vi "FreshTableDisplay.vi"(8 "error in (no error)":errorcluster, 10 "IndexDelta":i32, 11 "AdvanceTable in":refnum<class "AdvanceTable.lvclass">) -> (0 "error out":errorcluster, 3 "AdvanceTable out":refnum<class "AdvanceTable.lvclass">)   [LabVIEW 2015, in "ActorManagement.lvlib" / "AdvanceTable.lvclass"]
uses:
  AdvanceTable.lvclass
  AdvanceTable.lvclass/AdvanceTable.ctl
  Config/g_tabSetting.vi
  ActorManagement.lvlib
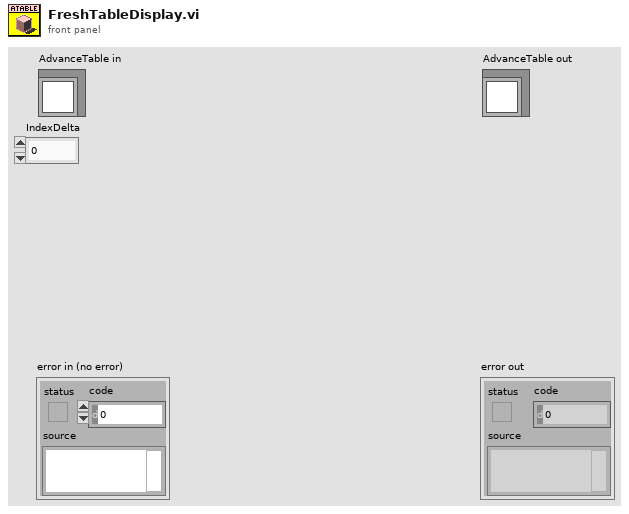
[diagram p1: front panel]
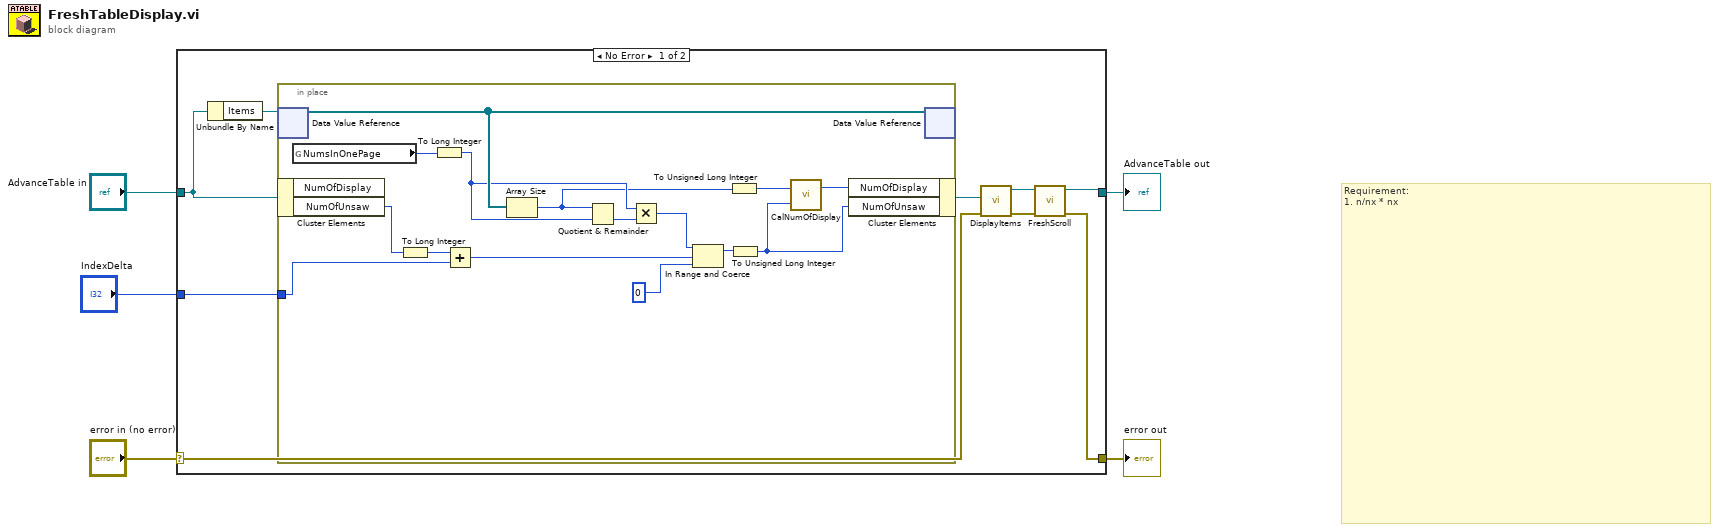
[diagram p0: block diagram]
diagram:
  # "Requirement:\n1. n/nx * nx"
  n1 = case shown="No Error" "error in (no error)" {
    selector: "error in (no error)" -> [w10 w31]
    tunnel: [w7 w31] -> w4
    tunnel: [w6 w30] -> w2
    tunnel: "AdvanceTable in" -> [w13 w30]
    tunnel: "IndexDelta" -> [w14 _]
    frame No Error {
      n2 = Unbundle By Name(w13) -> ("Items"=w12:refnum<data-value>)
      n3 = in-place {
        in-place-border: w14 -> [w26]
        n4 = in-place-dvr #1(w12) -> (w27:refnum<class "TableItem.lvclass">[])  [unwired: 1 out]
        n5 = in-place-cluster #2(w13) -> ("NumOfUnsaw"=w24:u32)  [unwired: 1 out]
        n6 = global read "g_tabSetting.vi" "NumsInOnePage"() -> (w21:u32)
        n7 = To Long Integer(number=w24) -> (32bit integer=w23:i32)
        n8 = To Long Integer(number=w21) -> (32bit integer=w20:i32)
        n9 = Add(x=w23, y=w26) -> (x+y=w22:i32)
        n10 = Array Size(array=w27) -> (size(s)=w16:i32)
        n11 = Quotient & Remainder(x=w16, y=w20) -> (floor(x/y)=w28:i32)  [unwired: 1 out]
        n12 = Multiply(x=w20, y=w28) -> (x*y=w19:i32)
        n13 = In Range and Coerce(upper limit=w19, x=w22, lower limit=0) -> (coerced(x)=w18:i32)  [unwired: 1 out]
        n14 = To Unsigned Long Integer(number=w16) -> (unsigned 32bit integer=w17:u32)
        n15 = To Unsigned Long Integer(number=w18) -> (unsigned 32bit integer=w15:u32)
        n16 = call "CalNumOfDisplay.vi"("IndexOfBase"=w15, "DataSum"=w17) -> ("NumOfDisplay"=w25:u32)  [unwired: 1 in]
        n17 = in-place-cluster #2("NumOfDisplay"=w25, "NumOfUnsaw"=w15) -> (w11:refnum<class "AdvanceTable.lvclass">)
        n18 = in-place-dvr #1(w27) -> ()  [unwired: 2 out]
      }
      n19 = call "DisplayItems.vi"("error in (no error)"=w10, "AdvanceTable in"=w11) -> ("error out"=w8:errorcluster, "AdvanceTable out"=w9:refnum<class "AdvanceTable.lvclass">)  [unwired: 8 in]
      n20 = call "FreshScroll.vi"("error in (no error)"=w8, "AdvanceTable in"=w9) -> ("error out"=w7:errorcluster, "AdvanceTable out"=w6:refnum<class "AdvanceTable.lvclass">)  [unwired: 8 in]
    }
    frame Error {
    }
  }
  "error out" <- w4
  "AdvanceTable out" <- w2
